vi "Write Span.vi"(8 "error in (no error)":errorcluster, 10 "Span":string, 11 "RxBN dBmHz Calculation in":refnum<class "RxBN dBmHz Calculation.lvclass">=refnum) -> (0 "error out":errorcluster, 3 "RxBN dBmHz Calculation out":refnum<class "RxBN dBmHz Calculation.lvclass">)   [LabVIEW 2016, in "SeqAuto Evaluations.lvlib" / "RxBN dBmHz Calculation.lvclass"]
uses:
  RxBN dBmHz Calculation.lvclass
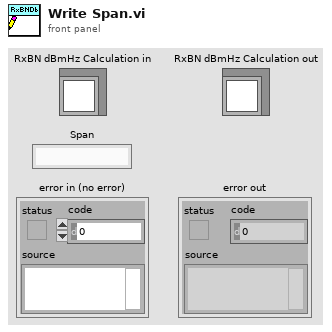
[diagram p1: front panel]
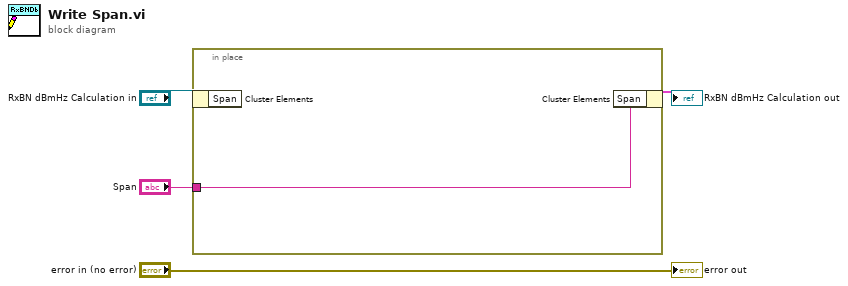
[diagram p0: block diagram]
diagram:
  n1 = in-place {
    in-place-border: "Span" -> [w5]
    n2 = in-place-cluster #1("RxBN dBmHz Calculation in") -> ()  [unwired: 1 out]
    n3 = in-place-cluster #1("Span"=w5) -> (→"RxBN dBmHz Calculation out":cluster{})
  }
  "error out" <- "error in (no error)"
